vi "test-diff-drive-odom-2-Test1.vi"() -> (3 "All Passed":bool)   [LabVIEW 2019]
uses:
  <vilib>/Rock Robotics/WPI/ThirdParty/JAS_Junk/TrajLib/VI/Quaternion_New.vi
  <vilib>/Rock Robotics/WPI/ThirdParty/JAS_Junk/TrajLib/VI/Translation3d_Create.vi
  <vilib>/Rock Robotics/WPI/ThirdParty/JAS_Junk/TrajLib/VI/Pose3d_New_Trans3dRot3d.vi
  <vilib>/Rock Robotics/WPI/ThirdParty/JAS_Junk/TrajLib/VI/AprilTag_GetAll.vi
  <vilib>/Rock Robotics/WPI/ThirdParty/JAS_Junk/TrajLib/Trajectory_Library.lvlib
  <vilib>/Rock Robotics/WPI/ThirdParty/JAS_Junk/TrajLib/TypeDef/TRANSLATION2D.ctl
  <vilib>/Rock Robotics/WPI/ThirdParty/JAS_Junk/TrajLib/TypeDef/ROTATION2D.ctl
  <vilib>/Rock Robotics/WPI/ThirdParty/JAS_Junk/TrajLib/TypeDef/POSE2D.ctl
panel:
  out "Test 1 passed":bool
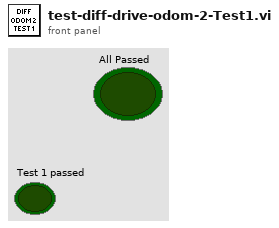
[diagram p1: front panel]
types:
  T1 = typedef "Trajectory_Library.lvlib/POSE2D.ctl" = cluster{"TRANSLATION":T2, "ROTATION":T3}
  T2 = typedef "Trajectory_Library.lvlib/TRANSLATION2D.ctl" = cluster{"X":dbl, "Y":dbl}
  T3 = typedef "Trajectory_Library.lvlib/ROTATION2D.ctl" = cluster{"VALUE":dbl, "COS":dbl, "SIN":dbl}
  T4 = typedef "Trajectory_Library.lvlib/DIFF_DRIVE_ODOM2.ctl" = cluster{"M_POSE_Meters":T1, "M_GyroOffset":T3, "M_PrevAngle":T3, "M_PrevLeftDist_M":dbl, "M_PrevRightDist_M":dbl, "M_InitLeftDist_M":dbl, "M_InitRightDist_M":dbl}
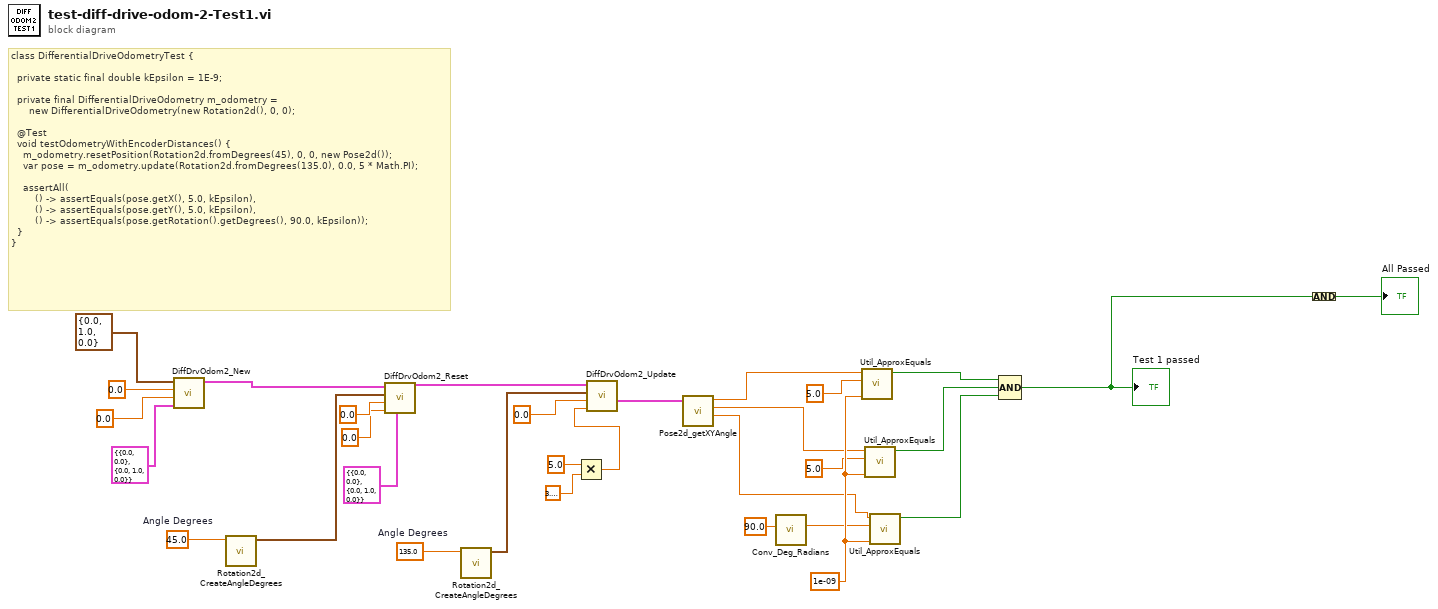
[diagram p0: block diagram]
diagram:
  w12 = 1e-09 ("Tolerance")
  w19 = 135.0  # Angle Degrees
  w25 = 45.0  # Angle Degrees
  # "class DifferentialDriveOdometryTest {\n\n  private static final double kEpsilon = 1E-9;\n\n  private final DifferentialDriveOdometry m_odometry =\n      new DifferentialDriveOdometry(new Rotation2d(), 0, 0);\n\n  @Test\n  void testOdometryWithEncoderDistances() {\n    m_odometry.resetPosition(Rotation2d.fromDegrees(45), 0, 0, new Pose2d());\n    var pose = m_odometry.update(Rotation2d.fromDegrees(135.0), 0.0, 5 * Math.PI);\n\n    assertAll(\n        () -> assertEquals(pose.getX(), 5.0, kEpsilon),\n        () -> assertEquals(pose.getY(), 5.0, kEpsilon),\n        () -> assertEquals(pose.getRotation().getDegrees(), 90.0, kEpsilon));\n  }\n}"
  n1 = call <vilib>:"DiffDrvOdom2_New.vi"("Initial Pose Meters"=T1 {"TRANSLATION"={"X"=0.0, "Y"=0.0}, "ROTATION"={"VALUE"=0.0, "COS"=1.0, "SIN"=0.0}}, "Initial Right Distance M"=0.0, "Initial Left Distance M"=0.0, "Initial Gyro Reading"=T3 {"VALUE"=0.0, "COS"=1.0, "SIN"=0.0}) -> ("Out DIFF_DRIVE_ODOM"=w26:T4)  [unwired: 7 in]
  n2 = call <vilib>:"Rotation2d_CreateAngleDegrees.vi"("Angle_Degrees"=w25) -> ("ROTATION"=w24:T3)  [unwired: 10 in]
  n3 = call <vilib>:"DiffDrvOdom2_Reset.vi"("Pose Meters"=T1 {"TRANSLATION"={"X"=0.0, "Y"=0.0}, "ROTATION"={"VALUE"=0.0, "COS"=1.0, "SIN"=0.0}}, "Right Distance M"=0.0, "Left Distance M"=0.0, "Gyro Reading"=w24, "In DIFF_DRIVE_ODOM"=w26) -> ("Out DIFF_DRIVE_ODOM"=w20:T4)  [unwired: 6 in]
  n4 = call <vilib>:"Rotation2d_CreateAngleDegrees.vi"("Angle_Degrees"=w19) -> ("ROTATION"=w18:T3)  [unwired: 10 in]
  n5 = Multiply(x=5.0, y=3.141592653589793) -> (x*y=w14:dbl)
  n6 = call <vilib>:"DiffDrvOdom2_Update.vi"("Right Distance M"=w14, "Left Distance M"=0.0, "Gyro Reading"=w18, "In DIFF_DRIVE_ODOM"=w20) -> ("Pose Meters"=w13:T1)  [unwired: 6 in, 1 out]
  n7 = call <vilib>:"Pose2d_getXYAngle.vi"("in POSE"=w13) -> ("Angle"=w7:dbl, "Y"=w10:dbl, "X"=w11:dbl)  [unwired: 8 in]
  n8 = call <vilib>:"Conv_Deg_Radians.vi"("Degress"=90.0) -> ("Radians"=w9:dbl)  [unwired: 10 in]
  n9 = call <vilib>:"Util_ApproxEquals.vi"("Tolerance"=w12, "Value 2"=5.0, "Value 1"=w11) -> ("ApproxEquals"=w4:bool)  [unwired: 8 in]
  n10 = call <vilib>:"Util_ApproxEquals.vi"("Tolerance"=w12, "Value 2"=5.0, "Value 1"=w10) -> ("ApproxEquals"=w3:bool)  [unwired: 8 in]
  n11 = call <vilib>:"Util_ApproxEquals.vi"("Tolerance"=w12, "Value 2"=w9, "Value 1"=w7) -> ("ApproxEquals"=w2:bool)  [unwired: 8 in]
  n12 = Compound Arithmetic op=AND(w4, w3, w2) -> (w1:bool)
  "Test 1 passed" <- w1
  n13 = Compound Arithmetic op=AND(w1) -> (→"All Passed":bool)
